vi "JSONInt64.vi"(9 "return":i64) -> (3 "JSON string":string)   [LabVIEW 2026]
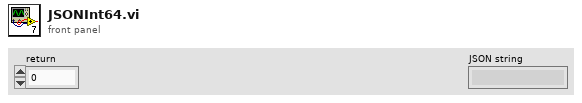
[diagram p1: front panel]
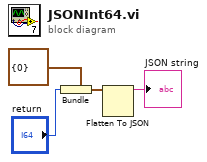
[diagram p0: block diagram]
diagram:
  n1 = Bundle(cluster=cluster{"return":i64} {"return"=0}, "return"="return") -> (w4:cluster{"return":i64})
  n2 = Flatten To JSON(anything=w4) -> (JSON string=→"JSON string":string)  [unwired: 2 in, 1 out]
